vi "Get Msg Queue Status__ogtk.vi"(8 "error in (no error)":errorcluster, 10 "return elements (F)":bool, 11 "msg queue":T3) -> (0 "error out":errorcluster, 1 "# pending to insert":i32, 2 "# pending to remove":i32, 3 "msg queue out":T3, 4 "# elements in queue":i32, 5 "name":string, 6 "messages":T1[](array[typedef]), 7 "queue size":i32)   [LabVIEW 2012]
doc: "Returns current status information of message queue."
uses:
  <userlib>/_OpenG.lib/msgqueue/msgqueue.llb/Msg Queue RefNum__ogtk.ctl
  <userlib>/_OpenG.lib/msgqueue/msgqueue.llb/Msg Cluster__ogtk.ctl
panel:
  # "[OpenG VI Tags] ***Do Not Remove***"
  # "Get Msg Queue Status.vi\n\nReturns current status information of message queue.\n\nPlease visit http://www.OpenG.org to learn about the\nOpen Source LabVIEW software movement.\n\nNOTICE -- YOU MUST LEAVE THIS NOTICE IN PLACE.  PER THE TERMS OF THE LICENSE BELOW, YOU MAY SUBLICENSE THIS SOFTWARE \nIN ANY WAY THAT DOES NOT CONFLICT WITH THIS LICENSE.\n\n### BSD License (http://www.opensource.org/licenses/bsd-license.php) Begin ###\n\nCopyright (c) 2002, Jim Kring <jim@jimkring.com>\n\nAll rights reserved.\n\nRedistribution and use in source and binary forms, with or without modification, are permitted provided that the following conditions are met:\n\n    * Redistributions of source code must retain the above copyright notice, this list of conditions and the following disclaimer.\n    * Redistributions in binary form must reproduce the above copyright notice, this list of conditions and the following disclaimer in the \n       documentation and/or other materials provided with the distribution.\n    * Neither the name of SciWare, James Kring, Inc., nor the names of its contributors may be used to endorse or promote products derived \n       from this software without specific prior written permission.\n\nTHIS SOFTWARE IS PROVIDED BY THE COPYRIGHT HOLDERS AND CONTRIBUTORS \"AS IS\" AND ANY EXPRESS OR IMPLIED WARRANTIES, \nINCLUDING, BUT NOT LIMITED TO, THE IMPLIED WARRANTIES OF MERCHANTABILITY AND FITNESS FOR A PARTICULAR PURPOSE ARE \nDISCLAIMED. IN NO EVENT SHALL THE COPYRIGHT OWNER OR CONTRIBUTORS BE LIABLE FOR ANY DIRECT, INDIRECT, INCIDENTAL,\n SPECIAL, EXEMPLARY, OR CONSEQUENTIAL DAMAGES (INCLUDING, BUT NOT LIMITED TO, PROCUREMENT OF SUBSTITUTE GOODS OR \nSERVICES; LOSS OF USE, DATA, OR PROFITS; OR BUSINESS INTERRUPTION) HOWEVER CAUSED AND ON ANY THEORY OF LIABILITY, \nWHETHER IN CONTRACT, STRICT LIABILITY, OR TORT (INCLUDING NEGLIGENCE OR OTHERWISE) ARISING IN ANY WAY OUT OF THE USE \nOF THIS SOFTWARE, EVEN IF ADVISED OF THE POSSIBILITY OF SUCH DAMAGE.\n\n### BSD License End ###"
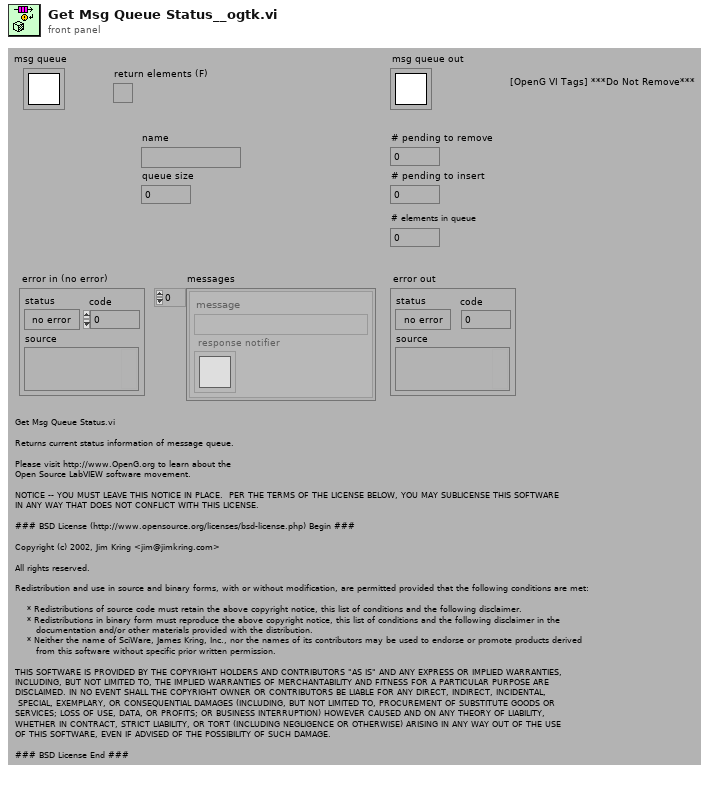
[diagram p1: front panel]
types:
  T1 = typedef "Msg Cluster__ogtk.ctl" = cluster{"message":string, "response notifier":T2}
  T2 = typedef "Notifier RefNum" = refnum<k1>
  T3 = typedef "Msg Queue RefNum__ogtk.ctl" = refnum<k1>
  T4 = typedef "Queue RefNum" = refnum<k1>
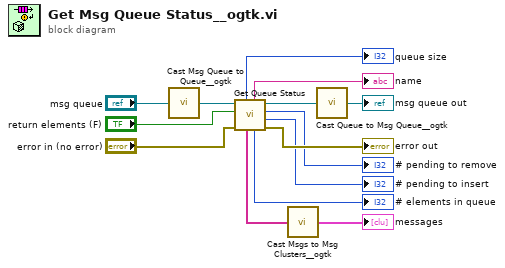
[diagram p0: block diagram]
diagram:
  n1 = call <userlib>:"Cast Msg Queue to Queue__ogtk.vi"("msg queue"="msg queue") -> ("queue"=w5:T4)  [unwired: 4 in]
  n2 = call <vilib>:"Get Queue Status.vi"("error in (no error)"="error in (no error)", "return elements (F)"="return elements (F)", "queue"=w5) -> ("error out"=→"error out":errorcluster, "# pending to insert"=→"# pending to insert":i32, "# pending to remove"=→"# pending to remove":i32, "queue out"=w4:T4, "# elements in queue"=→"# elements in queue":i32, "name"=→"name":string, "elements"=w2:string[], "queue size"=→"queue size":i32)  [unwired: 1 in]
  n3 = call <userlib>:"Cast Msgs to Msg Clusters__ogtk.vi"("queue elements"=w2) -> ("massages"=→"messages":T1[])  [unwired: 4 in]
  n4 = call <userlib>:"Cast Queue to Msg Queue__ogtk.vi"("queue"=w4) -> ("msg queue"=→"msg queue out":T3)  [unwired: 4 in]
